vi "Set Class Instance.vi"(8 "error in (no error)":errorcluster, 11 "Oscilloscope Model":string) -> (0 "error out":errorcluster, 3 "Oscilloscope":refnum<class "Oscilloscope.lvclass">)   [LabVIEW 2020, in "Oscilloscope VI.lvlib"]
uses:
  Oscilloscope VI/Oscilloscope VI.lvlib
  Oscilloscope.lvclass
  Scope 2 Test/Scope 2 Test.lvclass
  C:/Users/DELL/Documents/GitClones/Labview/OscilloscopeDQMH_OOP/Oscilloscope_DQMH_OOP/Libraries/Classes/Oscilloscope/Oscilloscope.lvclass
  Scope 1 Test/Scope 1 Test.lvclass
panel:
  out "class name":string
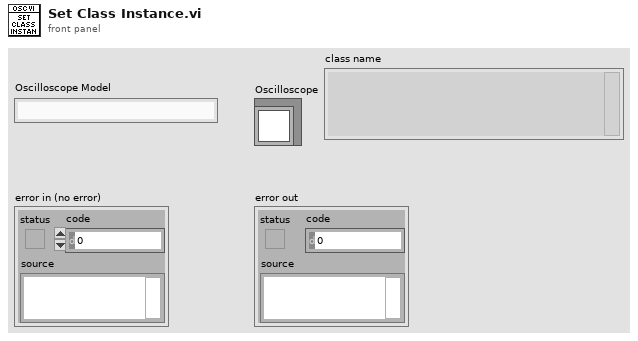
[diagram p1: front panel]
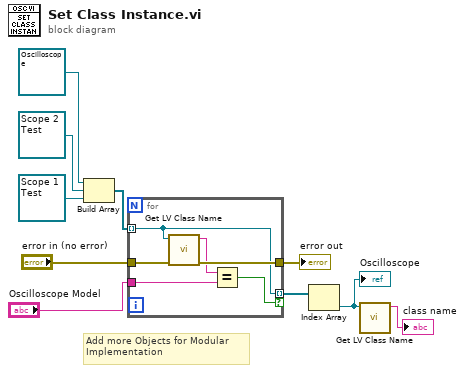
[diagram p0: block diagram]
diagram:
  # "Add more Objects for Modular\nImplementation"
  n1 = Build Array(refnum<class "Oscilloscope.lvclass"> refnum ("Oscilloscope VI.lvlib:Oscilloscope.lvclass"), refnum<class "Scope 2 Test.lvclass"> refnum ("Oscilloscope VI.lvlib:Scope 2 Test.lvclass"), refnum<class "Scope 1 Test.lvclass"> refnum ("Oscilloscope VI.lvlib:Scope 1 Test.lvclass")) -> (w9:refnum<class "Oscilloscope.lvclass">[])
  n2 = for {
    tunnel: w9 -> [w12] mode=indexing
    tunnel: "error in (no error)" -> [w16]
    tunnel: [w15] -> w7
    tunnel: "Oscilloscope Model" -> [w13]
    tunnel: [w12] -> w5 mode=indexing if=w11
    n3 = call <vilib>:"Get LV Class Name.vi"("error in (no error)"=w16, "object"=w12) -> ("error out"=w15:errorcluster, "class name"=w14:string)  [unwired: 8 in]
    n4 = Equal?(x=w14, y=w13) -> (x = y?=w11:bool)
  }
  "error out" <- w7
  n5 = Index Array(array=w5) -> (element=w2:refnum<class "Oscilloscope.lvclass">)  [unwired: 1 in]
  "Oscilloscope" <- w2
  n6 = call <vilib>:"Get LV Class Name.vi"("object"=w2) -> ("class name"=→"class name":string)  [unwired: 9 in, 1 out]
